vi "Queue Comms Flush Enqueue.vi"(8 "error in (no error)":errorcluster, 11 "element":T1) -> (0 "error out":errorcluster)   [LabVIEW 2018]
doc: "This subVI flushes the queue then enqueues an element in to the communications queue to be handled"
uses:
  Private Controls/Module Data.ctl
  Private Controls/Module Action.ctl
  Error Handler.lvlib
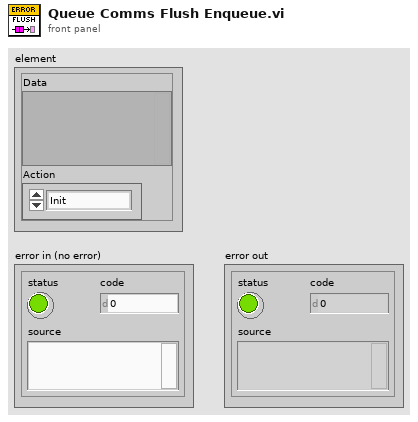
[diagram p1: front panel]
types:
  T1 = typedef "Error Handler.lvlib/Module Data.ctl" = cluster{"Data":variant, "Action":T2}
  T2 = typedef "Error Handler.lvlib/Module Action.ctl" = enum8{"Init", "Error", "Exit", "Module Error", "Controller Error", "User Interface Error", "File IO Error", "cRIO Error", "Calibration Error", "cRIO Health Alert", "FPGA Health Alert"}
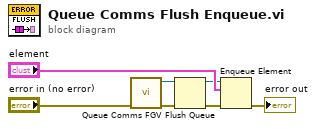
[diagram p0: block diagram]
diagram:
  n1 = call "Queue Comms FGV.vi"("error in (no error)"="error in (no error)") -> ("error out"=w2:errorcluster, "Queue out"=w5:refnum<queue>)  [unwired: 9 in]
  n2 = Flush Queue(queue=w5, error in (no error)=w2) -> (queue out=w3:refnum<queue>, error out=w1:errorcluster)  [unwired: 1 out]
  n3 = Enqueue Element(queue=w3, element="element", error in (no error)=w1) -> (error out=→"error out":errorcluster)  [unwired: 1 in, 2 out]
